vi "Log In 2.0.vi"(10 "required access level":i32, 11 "Program Root Path":path=path "C:/Labview Code") -> (0 "Password Out":string, 1 "User Name Out":string, 2 "Cancelled":bool, 3 "passed":bool)   [LabVIEW 2018]
panel:
  in  "User Name":string
  in  "Cancel":bool
  in  "Ok":bool
  in  "Password":string
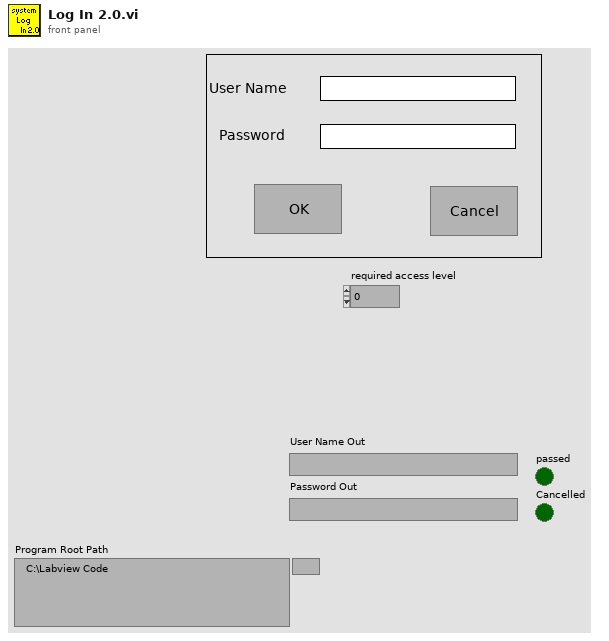
[diagram p1: front panel]
types:
  T1 = cluster{"Program Root Path":path, "Cancelled":bool, "Passed":bool, "User Names":string[], "Passwords":string[], "User Name Index":i32, "access levels":i32[]}
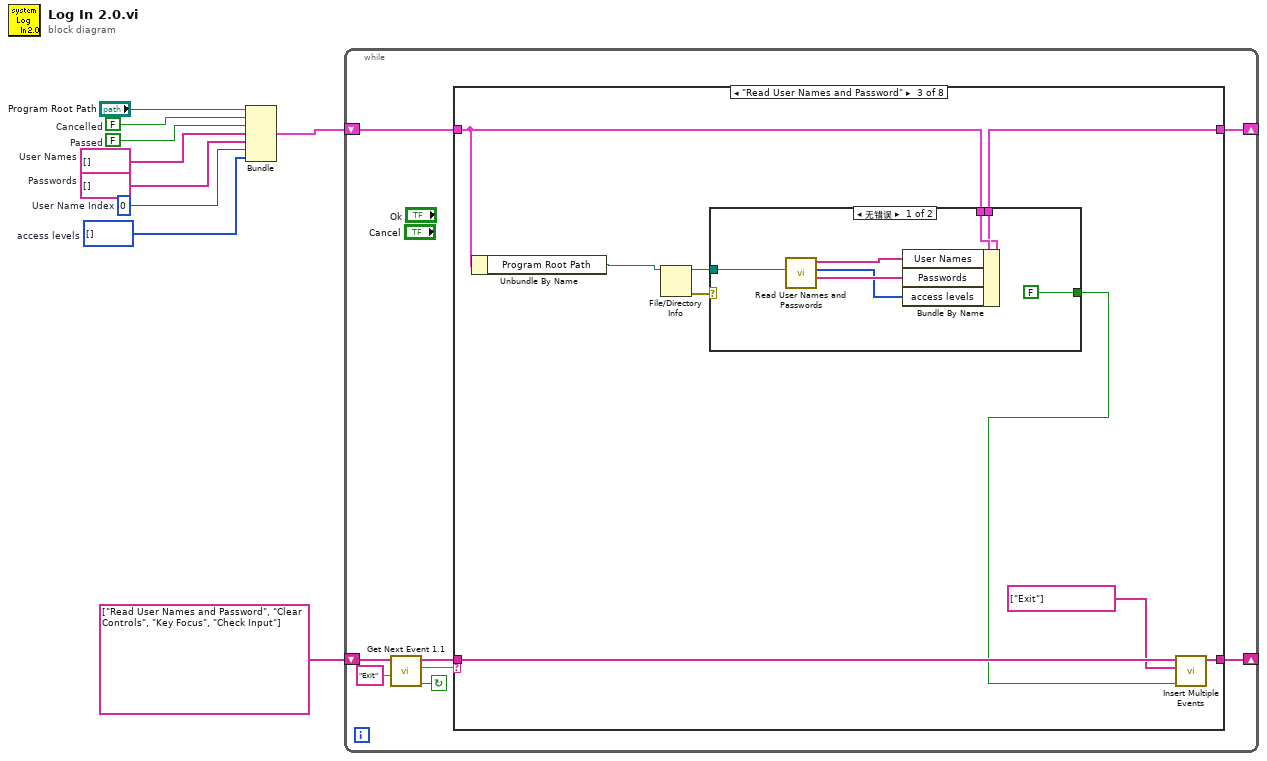
[diagram p0: block diagram]
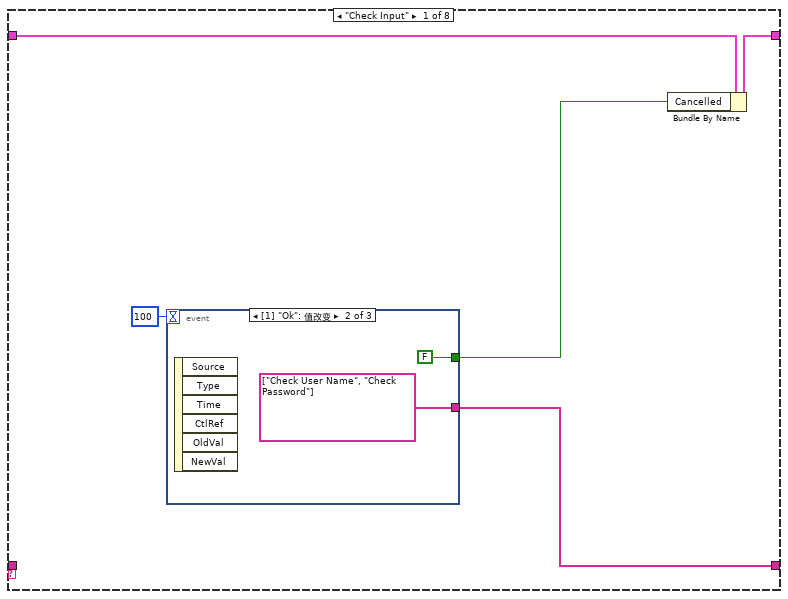
[diagram p2: hidden frame]
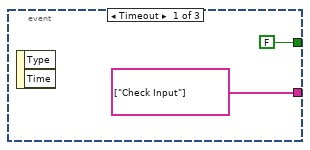
[diagram p3: hidden frame]
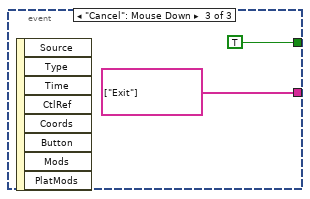
[diagram p4: hidden frame]
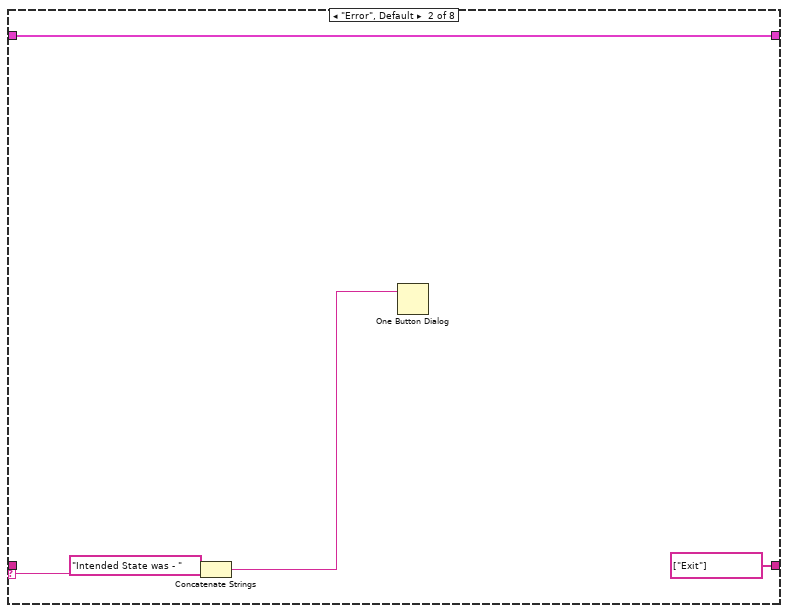
[diagram p5: hidden frame]
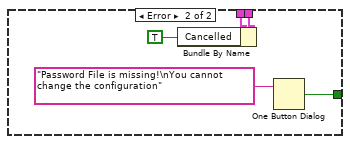
[diagram p6: hidden frame]
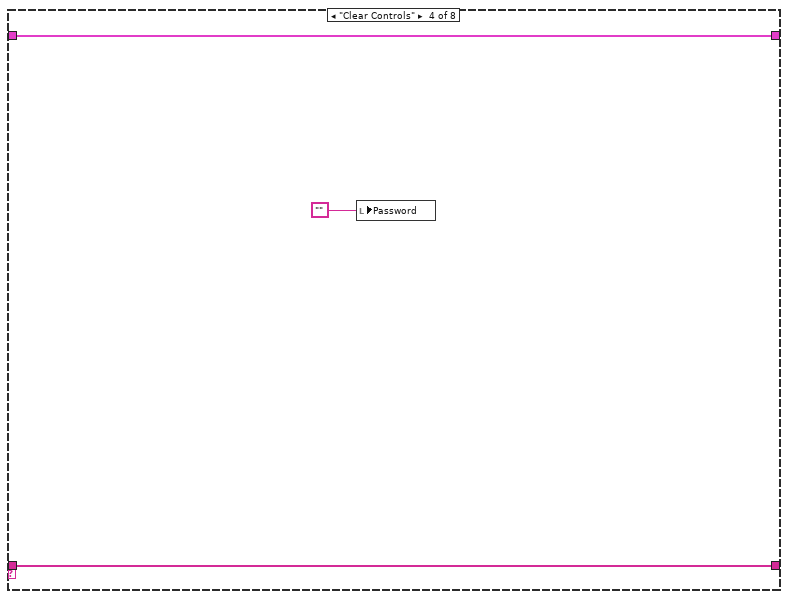
[diagram p7: hidden frame]
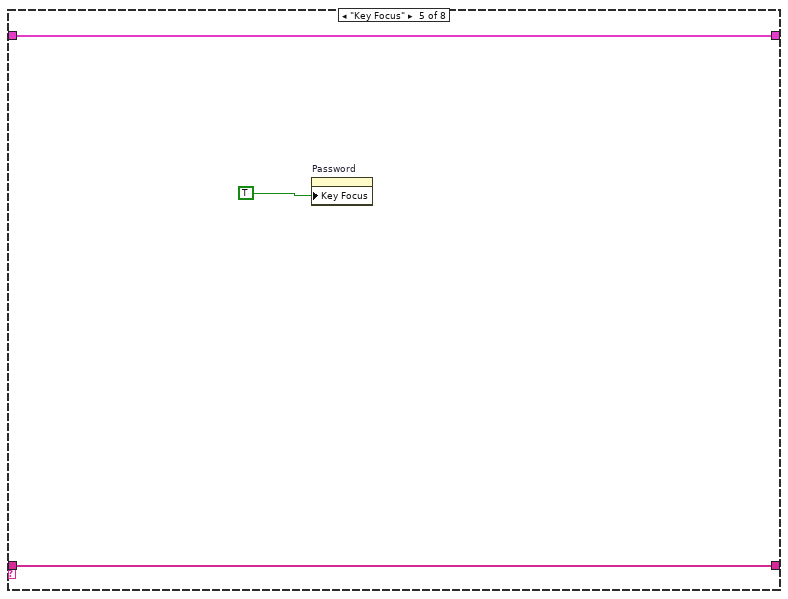
[diagram p8: hidden frame]
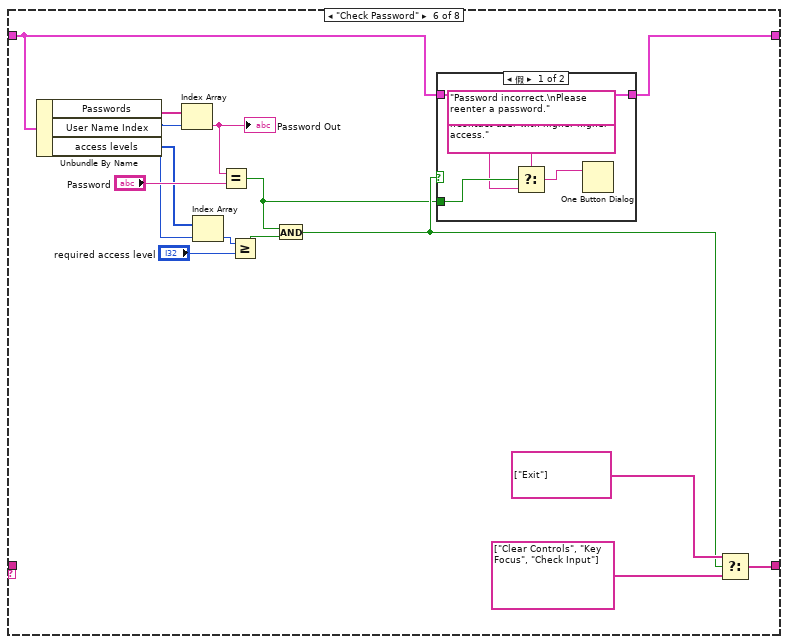
[diagram p9: hidden frame]
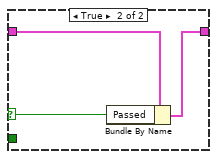
[diagram p10: hidden frame]
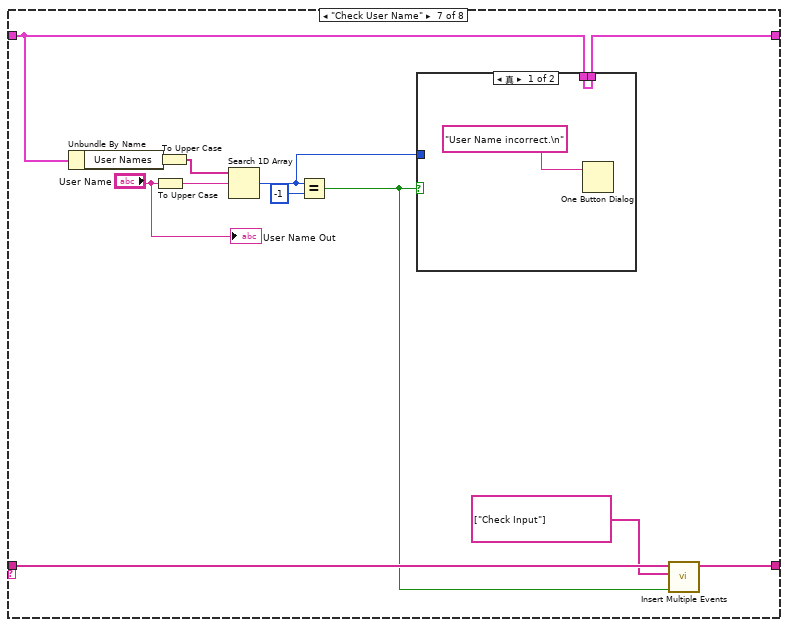
[diagram p11: hidden frame]
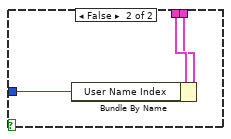
[diagram p12: hidden frame]
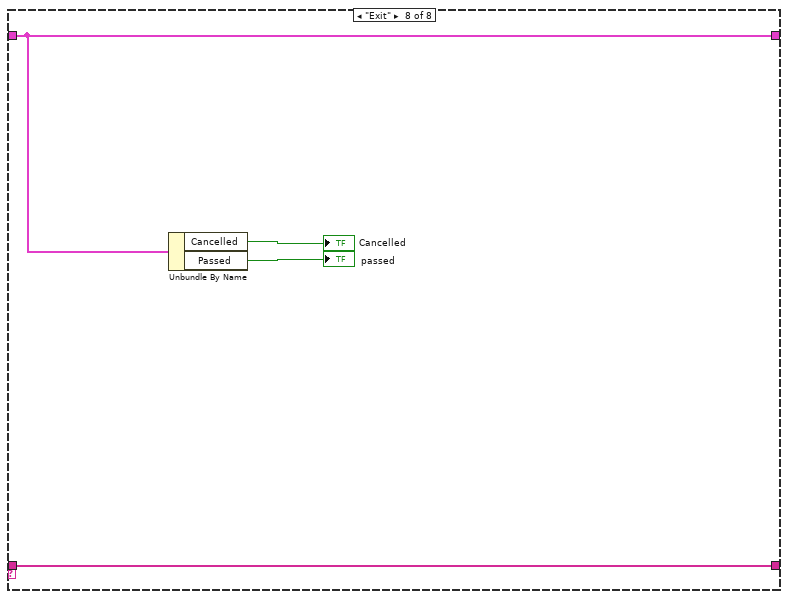
[diagram p13: hidden frame]
diagram:
  w1 = i32[] []  # access levels
  w2 = 0  # User Name Index
  w3 = string[] []  # User Names
  w4 = string[] []  # Passwords
  w5 = FALSE  # Passed
  w6 = FALSE  # Cancelled
  n1 = Bundle("Program Root Path"="Program Root Path", "Cancelled"=w6, "Passed"=w5, "User Names"=w3, "Passwords"=w4, "User Name Index"=w2, "access levels"=w1) -> (w7:T1)  [unwired: 1 in]
  n2 = while {
    shift-right: [w11] -> _
    shift-left: w7 -> [w12]
    shift-right: [w13] -> _
    shift-left: string[] ["Read User Names and Password", "Clear Controls", "Key Focus", "Check Input"] ("event queue out") -> [w15]
    stop <- w17 continue-if-true
    n3 = call "Get Next Event 1.1.vi"("Exit Event"="Exit", "event queue in"=w15) -> ("Condition (Exit:F)"=w17:bool, "next event"=w16:string, "event queue out"=w14:string[])  [unwired: 6 in, 1 out]
    n4 = case shown="\"Read User Names and Password\"" w16 {
      selector: w16 -> [_ w31 _ _ _ _ _ _]
      tunnel: [w20 string[] ["Exit"] ("event queue out") w38 w56 w60 w72 w87 w104] -> w13
      tunnel: w14 -> [_ _ w37 w56 w60 _ w86 w104]
      tunnel: w12 -> [w22 w32 w42 w57 w59 w74 w94 w103]
      tunnel: [w21 w32 w41 w57 w59 w75 w95 w103] -> w11
      frame "Check Input" {
        n5 = event shown="[1] \"Ok\": 值改变" {
          selector: _ -> [_ _ _]
          dyn-events: _ -> [_ _ _]
          timeout: 100 -> [_ _ _]
          tunnel: [string[] ["Check Input"] ("Events to Insert") string[] ["Check User Name", "Check Password"] ("Events to Insert") string[] ["Exit"] ("Events to Insert")] -> w20
          tunnel: [FALSE FALSE TRUE] -> w18
          event Timeout {
            n6 = event-data() -> ()  [unwired: 1 in, 2 out]
          }
          event "Ok": Value Change {
            n7 = event-data() -> ()  [unwired: 1 in, 6 out]
          }
          event "Cancel": Mouse Down {
            n8 = event-data() -> ()  [unwired: 1 in, 8 out]
          }
        }
        n9 = Bundle By Name(cluster=w22, "Cancelled"=w18) -> (w21:T1)
      }
      frame "Error", Default {
        n10 = Concatenate Strings("Intended State was - " ("string"), w31) -> (w30:string)
        n11 = One Button Dialog(message=w30) -> ()  [unwired: 1 in, 1 out]
      }
      frame "Read User Names and Password" {
        n12 = Unbundle By Name(w42) -> ("Program Root Path"=w34:path)
        n13 = File/Directory Info(path=w34) -> (path out=w39:path, error out=w40:errorcluster)  [unwired: 1 in, 5 out]
        n14 = case shown="无错误" w40 {
          tunnel: w42 -> [w49 w53]
          tunnel: [w48 w52] -> w41
          tunnel: w39 -> [w46 _]
          tunnel: [FALSE ("true") w50] -> w36
          frame No Error {
            n15 = call "Read User Names and Passwords.vi"("Base Path"=w46) -> ("Passwords"=w44:string[], "access levels"=w43:i32[], "User Names"=w45:string[])  [unwired: 8 in]
            n16 = Bundle By Name(cluster=w49, "User Names"=w45, "Passwords"=w44, "access levels"=w43) -> (w48:T1)
          }
          frame Error {
            n17 = Bundle By Name(cluster=w53, "Cancelled"=TRUE) -> (w52:T1)
            n18 = One Button Dialog(message="Password File is missing!\nYou cannot change the configuration") -> (true=w50:bool)  [unwired: 1 in]
          }
        }
        n19 = call "Insert Multiple Events.vi"("Insert all? (T)"=w36, "Events to Insert"=string[] ["Exit"], "Event queue in"=w37) -> ("Event queue out"=w38:string[])  [unwired: 4 in]
      }
      frame "Clear Controls" {
        n20 = local write "Password"("") -> ()
      }
      frame "Key Focus" {
        n21 = property on="Password" class="Str"("Key Focus"=TRUE) -> ()  [unwired: 2 in, 2 out]
      }
      frame "Check Password" {
        n22 = Unbundle By Name(w74) -> ("Passwords"=w69:string[], "User Name Index"=w66:i32, "access levels"=w67:i32[])
        n23 = Index Array(array=w69, index=w66) -> (element=w68:string)
        "Password Out" <- w68
        n24 = Index Array(array=w67, index=w66) -> (element=w65:i32)
        n25 = Equal?(x=w68, y="Password") -> (x = y?=w61:bool)
        n26 = Greater Or Equal?(x=w65, y="required access level") -> (x >= y?=w63:bool)
        n27 = And(x=w61, y=w63) -> (x .and. y?=w62:bool)
        n28 = case shown="假" w62 {
          selector: w62 -> [_ w81]
          tunnel: w74 -> [w80 w83]
          tunnel: [w80 w82] -> w75
          tunnel: w61 -> [w79 _]
          frame False {
            n29 = Select(t="Insufficient access level.\nContact user with higher higher access." ("message"), s=w79, f="Password incorrect.\nPlease reenter a password." ("message")) -> (s? t:f=w77:string)
            n30 = One Button Dialog(message=w77) -> ()  [unwired: 1 in, 1 out]
          }
          frame True {
            n31 = Bundle By Name(cluster=w83, "Passed"=w81) -> (w82:T1)
          }
        }
        n32 = Select(t=string[] ["Exit"] ("event queue out"), s=w62, f=string[] ["Clear Controls", "Key Focus", "Check Input"] ("event queue out")) -> (s? t:f=w72:string[])
      }
      frame "Check User Name" {
        n33 = Unbundle By Name(w94) -> ("User Names"=w93:string[])
        n34 = To Upper Case(1:"User Name") -> (0:w89:string)
        n35 = To Upper Case(1:w93) -> (0:w90:string[])
        n36 = Search 1D Array(1D array=w90, element=w89) -> (index of element=w91:i32)  [unwired: 1 in]
        n37 = Equal?(x=w91, y=-1) -> (x = y?=w85:bool)
        n38 = case shown="真" w85 {
          tunnel: w94 -> [w97 w100]
          tunnel: [w97 w99] -> w95
          tunnel: w91 -> [_ w98]
          frame True {
            n39 = One Button Dialog(message="User Name incorrect.\n") -> ()  [unwired: 1 in, 1 out]
          }
          frame False {
            n40 = Bundle By Name(cluster=w100, "User Name Index"=w98) -> (w99:T1)
          }
        }
        n41 = call "Insert Multiple Events.vi"("Insert all? (T)"=w85, "Events to Insert"=string[] ["Check Input"], "Event queue in"=w86) -> ("Event queue out"=w87:string[])  [unwired: 4 in]
        "User Name Out" <- "User Name"
      }
      frame "Exit" {
        n42 = Unbundle By Name(w103) -> ("Cancelled"=→"Cancelled":bool, "Passed"=→"passed":bool)
      }
    }
  }
